vi "Setup.vi"() -> ()   [LabVIEW 2013]
panel:
  in  "OK Button":bool
  in  "Comments":string
  in  "Cause":string(combo)
  in  "Furnace Interlock\n on data record":bool
  in  "Network Record":bool
  in  "Filename":string="Enter Filename"
  in  "Data Record":bool
  in  "Quench PID gains":T1={"proportional gain (Kc)"=-1.739, "integral time (Ti, min)"=28.69, "derivative time (Td, min)"=0.02} {"derivative time (Td, min)" format="%.3f"; "integral time (Ti, min)" format="%.3f"; "proportional gain (Kc)" format="%.3f"}
  in  "output range":cluster{"output high":dbl, "output low":dbl}={"output high"=80.0, "output low"=0.0} {"output low" format="%.2f"; "output high" format="%.2f"}
  out "output":dbl format="%.2f"
  out "TI-600 SP 2":dbl
  out "AI0":dbl
  in  "Use calculated Feed Rate\nin Conversion Calculation?":bool
  in  "Moist %":dbl=3.0
  in  "Biomass % Carbon":dbl=52.0
  in  "Inert particle %":dbl
  in  "O2 High Alarm\nV-600 & V-200":bool=TRUE
  in  "XV-200 Timed Operation":bool
  in  "SP (hrs)":dbl
  out "SP 2":dbl format="%<%H:%M:%S>t"
  in  "output range 2":cluster{"output high":dbl, "output low":dbl}={"output high"=100.0, "output low"=0.0} {"output low" format="%.2f"; "output high" format="%.2f"}
  in  "output range 3":cluster{"output high":dbl, "output low":dbl}={"output high"=20.0, "output low"=0.0} {"output low" format="%.2f"; "output high" format="%.2f"}
  in  "Steam boiler PID gains":T1={"proportional gain (Kc)"=1.778, "integral time (Ti, min)"=2.347, "derivative time (Td, min)"=0.222} {"derivative time (Td, min)" format="%.3f"; "integral time (Ti, min)" format="%.3f"; "proportional gain (Kc)" format="%.3f"}
  in  "Superheater PID gains":T1={"proportional gain (Kc)"=0.019, "integral time (Ti, min)"=0.9, "derivative time (Td, min)"=0.0129} {"derivative time (Td, min)" format="%.3f"; "integral time (Ti, min)" format="%.3f"; "proportional gain (Kc)" format="%.3f"}
  out "output 2":dbl format="%.2f"
  out "output 3":dbl format="%.2f"
  in  "Feed Rate to use":dbl=8.11
  out "Down event time":string
  out "Downtime":string caption="Elapsed Time Text"
  out "Uptime":string caption="Elapsed Time Text"
  in  "PCV-641 PID gains up":T1={"proportional gain (Kc)"=3.956, "integral time (Ti, min)"=13.06, "derivative time (Td, min)"=0.05} {"derivative time (Td, min)" format="%.3f"; "integral time (Ti, min)" format="%.3f"; "proportional gain (Kc)" format="%.3f"}
  in  "output range 5":cluster{"output high":dbl, "output low":dbl}={"output high"=0.0, "output low"=100.0}
  in  "output range 6":cluster{"output high":dbl, "output low":dbl}={"output high"=100.0, "output low"=0.0} {"output low" format="%.2f"; "output high" format="%.2f"}
  in  "Steam boiler PID gains 2":T1={"proportional gain (Kc)"=1.778, "integral time (Ti, min)"=2.347, "derivative time (Td, min)"=0.222} {"derivative time (Td, min)" format="%.3f"; "integral time (Ti, min)" format="%.3f"; "proportional gain (Kc)" format="%.3f"}
  out "Output 4":dbl format="%#_4g"
  in  "XV-201 Interlock":bool=TRUE
  in  "Feeder PID gains":T1={"proportional gain (Kc)"=1.231, "integral time (Ti, min)"=2.841, "derivative time (Td, min)"=0.055} {"derivative time (Td, min)" format="%.3f"; "integral time (Ti, min)" format="%.3f"; "proportional gain (Kc)" format="%.3f"}
  in  "output range 7":cluster{"output high":dbl, "output low":dbl}={"output high"=22.0, "output low"=1.0} {"output low" format="%.2f"; "output high" format="%.2f"}
  in  "PCV-641 PID gains small down":T1={"proportional gain (Kc)"=3.968, "integral time (Ti, min)"=13.09, "derivative time (Td, min)"=0.05} {"derivative time (Td, min)" format="%.3f"; "integral time (Ti, min)" format="%.3f"; "proportional gain (Kc)" format="%.3f"}
  in  "P dif":dbl=2.0
  in  "PCV-641 PID gains large down":T1={"proportional gain (Kc)"=0.444, "integral time (Ti, min)"=2.0, "derivative time (Td, min)"=0.0} {"derivative time (Td, min)" format="%.3f"; "integral time (Ti, min)" format="%.3f"; "proportional gain (Kc)" format="%.3f"}
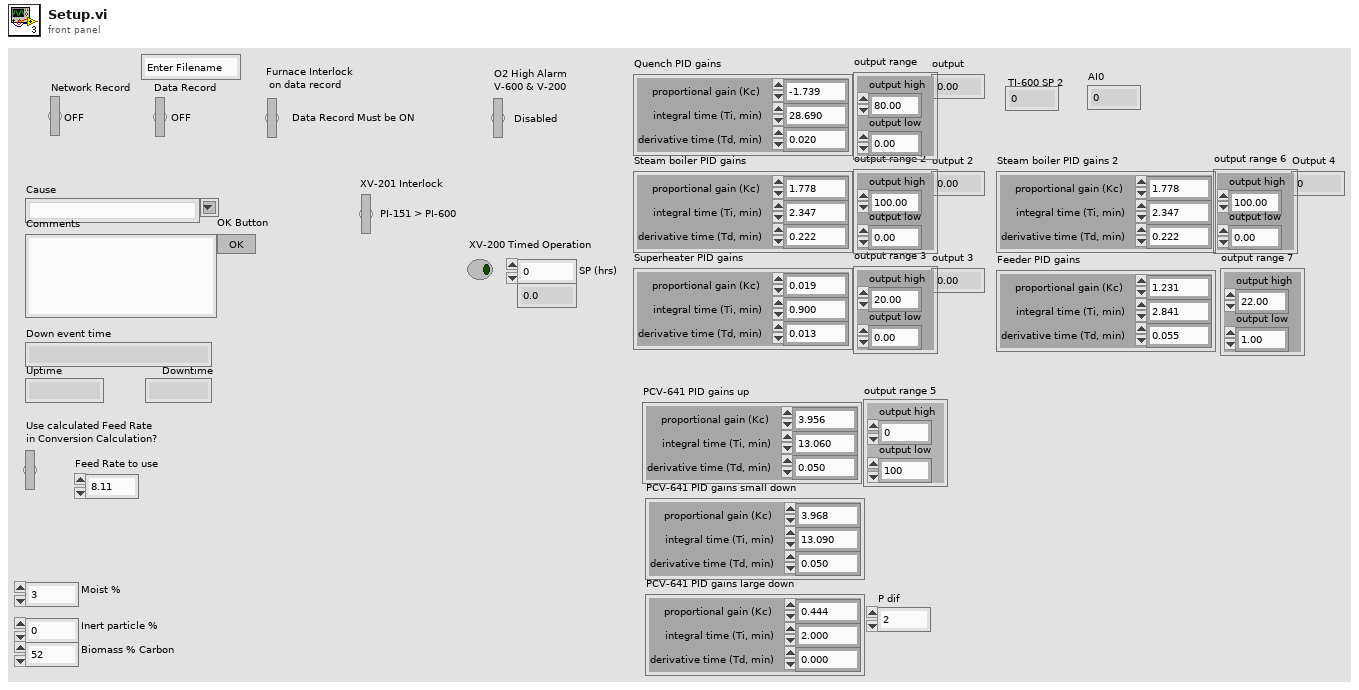
[diagram p1: front panel]
types:
  T1 = cluster{"proportional gain (Kc)":dbl, "integral time (Ti, min)":dbl, "derivative time (Td, min)":dbl}
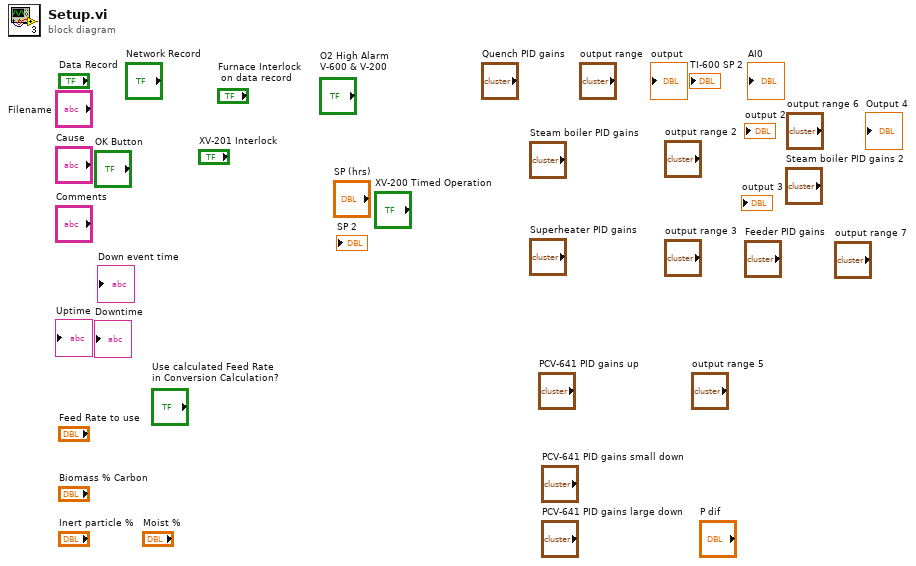
[diagram p0: block diagram]
diagram:
